vi "LVIS_Event.vi"(8 "Error In":errorcluster, 11 "EventInfo":T1) -> (0 "Error Out":errorcluster)   [LabVIEW 2015]
doc: "Determines the Event Info based on the LVIS_Settings file and passed in values, giving precedence to the file and deriving values where requested. Validates all event data and clears the event log."
uses:
  Sub VIs/Globals/LVIS_IsGlobal.vi
  Sub VIs/Globals/LVIS_DcGlobals.vi
panel:
  out "DateTime":string
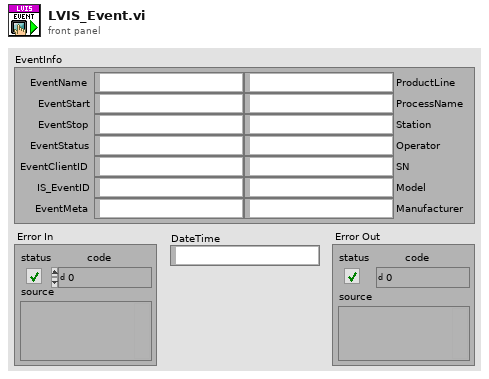
[diagram p1: front panel]
types:
  T1 = cluster{"EventName":string, "EventStart":string, "EventStop":string, "EventStatus":string, "EventClientID":string, "IS_EventID":string, "EventMeta":string, "ProductLine":string, "ProcessName":string, "Station":string, "Operator":string, "SN":string, "Model":string, "Manufacturer":string}
  T2 = cluster{"EventInfo":cluster{"EventName":string, "EventStart":string, "EventStop":string, "EventStatus":string, "EventClientID":string, "IS_EventID":string, "EventMeta":string, "ProductLine":string, "ProcessName":string, "Station":string, "Operator":string, "SN":string, "Model":string, "Manufacturer":string}, "TestInfo":cluster{"TestName":string, "TestDateTime":string, "TestStatus":string, "TestClientID":string, "IS_TestID":string, "TestMeta":string}, "MeasInfo":cluster{"MeasName":string, "MeasDateTime":string, "MeasStatus":string, "MeasClientID":string, "IS_MeasID":string, "MeasType":string, "MeasValue":string, "LL":string, "LL Comp":string, "HL":string, "HL Comp":string, "Units":string, "MeasMeta":string}}[]
  T3 = cluster{"[0]":string, "[1]":string, "[2]":string, "[3]":string, "[4]":string, "[5]":string, "[6]":string, "[7]":string, "[8]":string, "[9]":string, "[10]":string, "[11]":string, "[12]":string, "[13]":string}
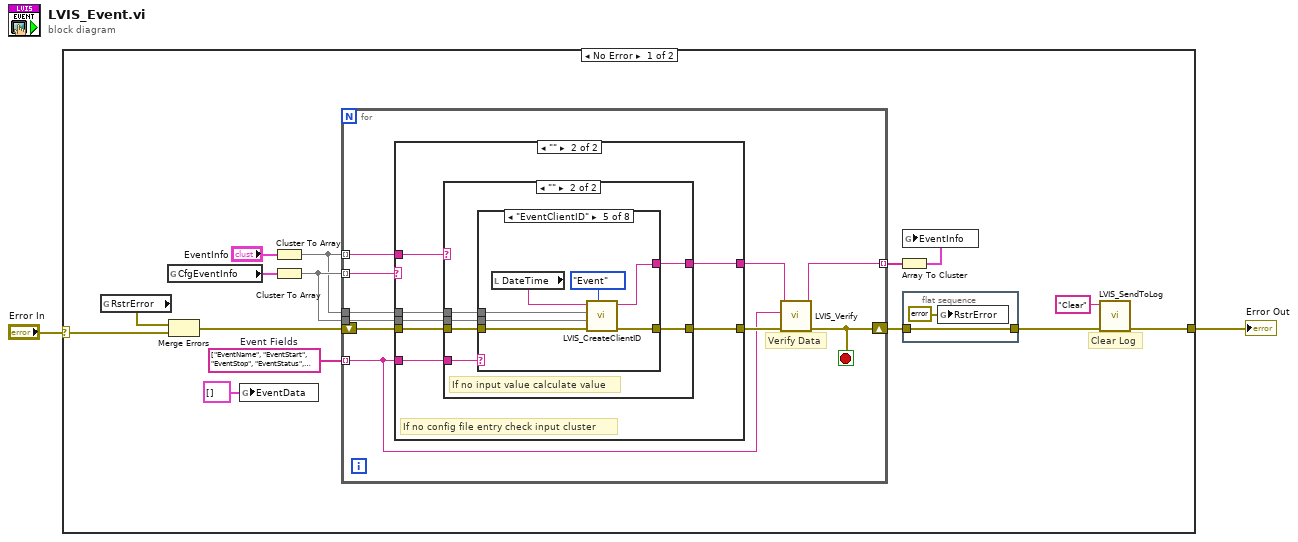
[diagram p0: block diagram]
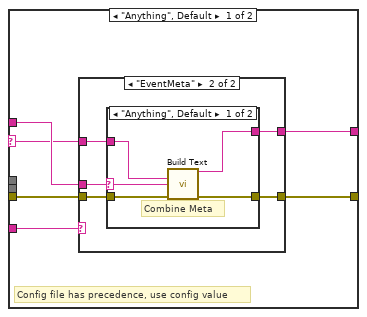
[diagram p2: hidden frame]
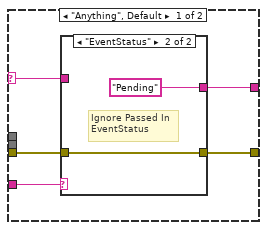
[diagram p5: hidden frame]
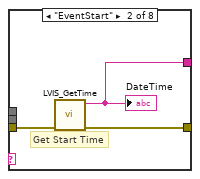
[diagram p8: hidden frame]
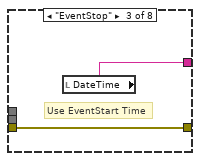
[diagram p9: hidden frame]
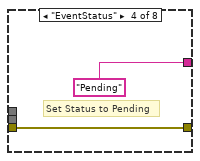
[diagram p10: hidden frame]
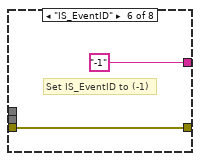
[diagram p11: hidden frame]
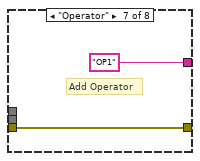
[diagram p12: hidden frame]
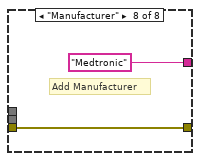
[diagram p13: hidden frame]
diagram:
  n1 = case shown="No Error" "Error In" {
    selector: "Error In" -> [w17 w93]
    tunnel: [w4 w93] -> w2
    frame No Error {
      w12 = string[] ["EventName", "EventStart", "EventStop", "EventStatus", "EventClientID", "IS_EventID", "EventMeta", "ProductLine", "ProcessName", "Station", "Operator", "SN", "Model", "Manufacturer"]  # Event Fields
      # "Clear Log"
      n2 = global read "LVIS_DcGlobals.vi" "RstrError"() -> (w8:errorcluster)
      n3 = global read "LVIS_IsGlobal.vi" "CfgEventInfo"() -> (w16:T1)
      n4 = Merge Errors(w8, w17) -> (w7:errorcluster)
      n5 = global write "LVIS_IsGlobal.vi" "EventData"(T2 [] ("EventData")) -> ()
      n6 = Cluster To Array(cluster="EventInfo") -> (array=w9:string[])
      n7 = Cluster To Array(cluster=w16) -> (array=w10:string[])
      n8 = for {
        tunnel: w10 -> [w24] mode=indexing
        tunnel: w12 -> [w22] mode=indexing
        shift-right: [w27] -> w6
        shift-left: w7 -> [w29]
        tunnel: w9 -> [w23] mode=indexing
        tunnel: [w25] -> w14 mode=indexing
        tunnel: w10 -> [w21]
        tunnel: w9 -> [w20]
        stop <- w27 stop-if-true
        # "Verify Data"
        n9 = case shown="\"\"" w24 {
          selector: w24 -> [w30 _]
          tunnel: w29 -> [w34 w55]
          tunnel: [w33 w54] -> w28
          tunnel: [w31 w53] -> w26
          tunnel: w22 -> [w35 w52]
          tunnel: w23 -> [w32 w56]
          tunnel: w21 -> [_ w51]
          tunnel: w20 -> [_ w50]
          frame "Anything", Default {
            # "Config file has precedence, use config value"
            n10 = case shown="\"EventMeta\"" w35 {
              tunnel: w34 -> [w37 w42]
              tunnel: [w37 w41] -> w33
              tunnel: w32 -> [_ w39]
              tunnel: [w36 w40] -> w31
              tunnel: w30 -> [w36 w38]
              frame "Other", Default {
                # "Non-Meta Config Data"
              }
              frame "EventMeta" {
                n11 = case shown="\"Anything\", Default" w39 {
                  selector: w39 -> [w44 _]
                  tunnel: w42 -> [w47 w48]
                  tunnel: [w46 w48] -> w41
                  tunnel: [w45 w49] -> w40
                  tunnel: w38 -> [w43 w49]
                  frame "Anything", Default {
                    # "Combine Meta"
                    n12 = call "Build Text"("Meta1"=w43, "Meta2"=w44, "error in (no error)"=w47) -> ("Result"=w45:string, "error out"=w46:errorcluster)  [unwired: 11 in]
                  }
                  frame "" {
                    # "No passed in Meta"
                  }
                }
              }
            }
          }
          frame "" {
            # "If no config file entry check input cluster"
            n13 = case shown="\"\"" w56 {
              selector: w56 -> [w60 _]
              tunnel: w55 -> [w58 w71]
              tunnel: [w57 w69] -> w54
              tunnel: [w59 w68] -> w53
              tunnel: w52 -> [w61 w70]
              tunnel: w51 -> [_ w67]
              tunnel: w50 -> [_ w66]
              frame "Anything", Default {
                n14 = case shown="\"EventStatus\"" w61 {
                  tunnel: w60 -> [w62 _]
                  tunnel: [w62 "Pending"] -> w59
                  tunnel: w58 -> [w63 w65]
                  tunnel: [w63 w65] -> w57
                  frame "Anything", Default {
                    # "Use Input Data\nif config empty"
                  }
                  frame "EventStatus" {
                    # "Ignore Passed In\nEventStatus"
                  }
                }
              }
              frame "" {
                # "If no input value calculate value"
                n15 = case shown="\"EventClientID\"" w70 {
                  tunnel: w71 -> [w72 w75 w77 w79 w86 w87 w89 w91]
                  tunnel: [w72 w74 w77 w79 w85 w87 w89 w91] -> w69
                  tunnel: [_ w73 w76 "Pending" ("Result") w80 "-1" ("ClientID") "OP1" ("ClientID") "Medtronic" ("ClientID")] -> w68
                  tunnel: w67 -> [_ _ _ _ w83 _ _ _]
                  tunnel: w66 -> [_ _ _ _ w82 _ _ _]
                  frame "Other", Default {
                    # "Value is not calculated"
                  }
                  frame "EventStart" {
                    # "Get Start Time"
                    n16 = call "LVIS_GetTime.vi"("Error In"=w75) -> ("Error out"=w74:errorcluster, "DateTime"=w73:string)  [unwired: 9 in]
                    "DateTime" <- w73
                  }
                  frame "EventStop" {
                    # "Use EventStart Time"
                    n17 = local read "DateTime"() -> (w76:string)
                  }
                  frame "EventStatus" {
                    # "Set Status to Pending"
                  }
                  frame "EventClientID" {
                    n18 = local read "DateTime"() -> (w84:string)
                    n19 = call "LVIS_CreateClientID.vi"("Type"=enum16{"Event", "Test", "Meas"}."Event", "Error In"=w86, "CfgInfo"=w83, "InputInfo"=w82, "DateTime"=w84) -> ("Error out"=w85:errorcluster, "ClientID"=w80:string)  [unwired: 5 in]
                  }
                  frame "IS_EventID" {
                    # "Set IS_EventID to (-1)"
                  }
                  frame "Operator" {
                    # "Add Operator"
                  }
                  frame "Manufacturer" {
                    # "Add Manufacturer"
                  }
                }
              }
            }
          }
        }
        n20 = call "LVIS_Verify.vi"("Error In"=w28, "Field Name"=w22, "Field Value In"=w26) -> ("Error Out"=w27:errorcluster, "Field Value Out"=w25:string)  [unwired: 7 in]
      }
      n21 = Array To Cluster(array=w14) -> (cluster=w13:T3)
      n22 = global write "LVIS_IsGlobal.vi" "EventInfo"(w13) -> ()
      n23 = flat-sequence {
        tunnel: w6 -> [w19]
        tunnel: [w19] -> w5
        frame #0 {
          n24 = global write "LVIS_DcGlobals.vi" "RstrError"(errorcluster {"status"=FALSE, "code"=0, "source"=""} ("RstrError")) -> ()
        }
      }
      n25 = call "LVIS_SendToLog.vi"("Error In"=w5, "EventData"="Clear") -> ("Error Out"=w4:errorcluster)  [unwired: 9 in]
    }
    frame Error {
    }
  }
  "Error Out" <- w2
